vi "SW_Type_1b_correction.vi"(1 "variable n":bool, 2 "wire diameter (mu.m)":dbl=5.0, 3 "calib consts. t2":dbl[](array[numeric]), 4 "calib consts. t1":dbl[](array[numeric])) -> (0 "Corrected calib consts. t2":dbl[](array[numeric]))   [LabVIEW 2010]
panel:
  # "Type 1b: Correct calibration constants at t2 to conditions at t1"
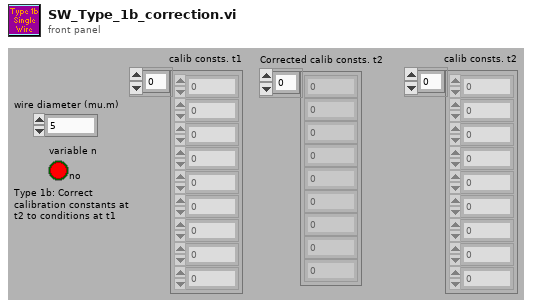
[diagram p1: front panel]
types:
  T1 = cluster{"calib consts. t1[0]":dbl, "calib consts. t1[1]":dbl, "calib consts. t1[2]":dbl, "calib consts. t1[3]":dbl, "calib consts. t1[4]":dbl, "calib consts. t1[5]":dbl, "calib consts. t1[6]":dbl, "calib consts. t1[7]":dbl}
  T2 = cluster{"calib consts. t2[0]":dbl, "calib consts. t2[1]":dbl, "calib consts. t2[2]":dbl, "calib consts. t2[3]":dbl, "calib consts. t2[4]":dbl, "calib consts. t2[5]":dbl, "calib consts. t2[6]":dbl, "calib consts. t2[7]":dbl}
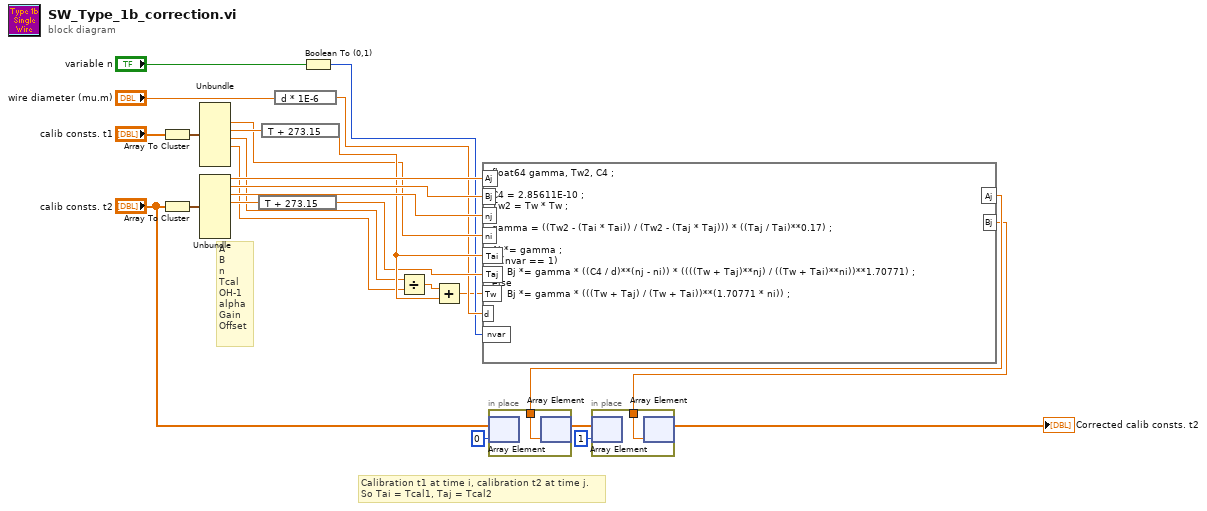
[diagram p0: block diagram]
diagram:
  # "Calibration t1 at time i, calibration t2 at time j.\nSo Tai = Tcal1, Taj = Tcal2"
  # "A\nB\nn\nTcal\nOH-1\nalpha\nGain\nOffset"
  n1 = Array To Cluster(array="calib consts. t1") -> (cluster=w17:T1)
  n2 = Array To Cluster(array="calib consts. t2") -> (cluster=w26:T2)
  n3 = Unbundle(w17) -> ("calib consts. t1[2]"=w13:dbl, "calib consts. t1[3]"=w15:dbl, "calib consts. t1[4]"=w14:dbl, "calib consts. t1[5]"=w1:dbl)  [unwired: 4 out]
  n4 = Unbundle(w26) -> ("calib consts. t2[0]"=w25:dbl, "calib consts. t2[1]"=w24:dbl, "calib consts. t2[2]"=w23:dbl, "calib consts. t2[3]"=w20:dbl)  [unwired: 4 out]
  n5 = expression code="T + 273.15"(w20) -> (w19:dbl)
  n6 = expression code="T + 273.15"(w15) -> (w21:dbl)
  n7 = expression code="d * 1E-6"("wire diameter (mu.m)") -> (w11:dbl)
  n8 = Boolean To (0,1)(Boolean="variable n") -> (0, 1=w9:i16)
  n9 = Divide(x=w14, y=w1) -> (x/y=w8:dbl)
  n10 = Add(x=w8, y=w21) -> (x+y=w7:dbl)
  n11 = formula code="float64 gamma, Tw2, C4 ;\n\nC4 = 2.85611E-10 ;\nTw2 = Tw * Tw ;\n\ngamma = ((Tw2 - (Tai * Tai)) / (Tw2 - (Taj * Taj))) * ((Taj / Tai)**0.17) ;\n\nAj *= gamma ;\nif (nvar == 1)\n     Bj *= gamma * ((C4 / d)**(nj - ni)) * ((((Tw + Taj)**nj) / ((Tw + Tai)**ni))**1.70771) ;\nelse\n     Bj *= gamma * (((Tw + Taj) / (Tw + Tai))**(1.70771 * ni)) ;"("Aj"=w25, "Bj"=w24, "nj"=w23, "Tai"=w21, "Taj"=w19, "Tw"=w7, "ni"=w13, "d"=w11, "nvar"=w9) -> ("Aj"=w5:dbl, "Bj"=w4:dbl)
  n12 = in-place {
    in-place-border: w5 -> [w27]
    n13 = in-place-array #1("calib consts. t2", 0) -> ()  [unwired: 1 out]
    n14 = in-place-array #1(w27) -> (w2:dbl[])  [unwired: 1 out]
  }
  n15 = in-place {
    in-place-border: w4 -> [w28]
    n16 = in-place-array #2(w2, 1) -> ()  [unwired: 1 out]
    n17 = in-place-array #2(w28) -> (→"Corrected calib consts. t2":dbl[])  [unwired: 1 out]
  }
